vi "OAT Overall Level Plot (1 Channel).vi"(0 "even-angle signal":cluster{"r0":dbl, "dr":dbl, "Y":dbl[]}={"r0"=0.0, "dr"=1.0, "Y"=[]} {"r0" format="%.2p"; "dr" format="%.2p"; "Y" format="%.2f"}, 1 "x-axis selection":u16(ring)=2 items=["Time", "Revolution", "RPM"], 2 "reset? (F)":bool, 5 "even-angle channel info":T3={"channel name"="", "description"="", " channel info"={"sensor sensitivity"=1000.0, "engineering units"=1, "dB reference"=1.0, "custom label"="EU", "weighting filter"=0, "pregain"=0.0}} {"channel info"."pregain" format="%.2f"; "channel info"."weighting filter" items=["Linear", "A-weighting", "B-weighting", "C-weighting", "ITU-R 468-4", "Dolby", "CCITT", "C-message", "Wb", "Wc", "Wd", "We", "Wf", "Wh", "Wj", "Wk", "Wm", "AES17 20 kHz lowpass", "AES17 40 kHz lowpass", "AES17 20 kHz highpass", "AES17 40 kHz highpass"]; "channel info"."dB reference" format="%^.1e"; "channel info"."engineering units" items=["custom..."=0, "V"=1, "A"=21, "C"=30, "pC"=31, "s"=32, "-"=29, "Pa"=2, "N"=20, "g"=3, "m/s^2"=4, "m/s"=5, "m"=6, "mm/s"=12, "mm"=13, "micron/s"=14, "micron"=15, "in/s^2"=7, "in/s"=8, "in"=9, "mil/s"=10, "mil"=11, "rad/s^2"=16, "rad/s"=17, "rad"=18, "deg/s^2"=26, "deg/s"=27, "deg"=28, "RPM"=22, "cycle/s^2"=23, "Hz"=24, "cycle"=25, "strain"=19]; "channel info"."sensor sensitivity" format="%#_5f"}, 7 "even-angle position info":T1, 9 "dB on? (F)":bool, 11 "error in (no error)":errorcluster, 12 "integration revolution":dbl=1.0) -> (4 "overall level":cluster{"time/rev/rpm":dbl[], "level":dbl[]}, 6 "unit labels":T2, 8 "level position info":T1, 15 "error out":errorcluster)   [LabVIEW 2017, in "SoundVib_OrderTracking.lvlib"]
doc: "Computes the root-mean-square (RMS) level of the <B>even-angle signal</B> and generates an XY graph as the output. Wire data to the <B>even-angle signal</B> input to determine the polymorphic instance to use or manually select the instance."
uses:
  <vilib>/addons/Sound and Vibration/Order Analysis/Resample Order Tracking/SoundVib_OrderTracking.lvlib
  <vilib>/addons/Sound and Vibration/Order Analysis/Misc/OAT Position Info.ctl
  <vilib>/addons/_NISVFA/_Shared subVIs/Controls/svc_Resampled Channel Info.ctl
  <vilib>/addons/_NISVFA/_Shared subVIs/Controls/svc_Channel Info.ctl
  <vilib>/addons/_NISVFA/_Shared subVIs/Controls/svc_Engineering Units Text Ring.ctl
  <vilib>/addons/_NISVFA/_Shared subVIs/Controls/svc_Weighting Filter Text Ring.ctl
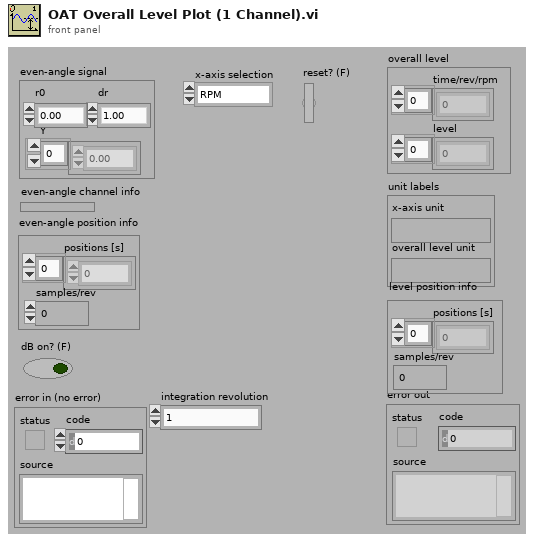
[diagram p1: front panel]
types:
  T1 = typedef "OAT Position Info.ctl" = cluster{"positions [s]":dbl[], "samples/rev":dbl}
  T2 = cluster{"x-axis unit":string, "overall level unit":string}
  T3 = typedef "svc_Resampled Channel Info.ctl" = cluster{"channel name":string, "description":string, " channel info":T4}
  T4 = typedef "svc_Channel Info.ctl" = cluster{"sensor sensitivity":dbl, "engineering units":T5, "dB reference":dbl, "custom label":string, "weighting filter":T6, "pregain":dbl}
  T5 = typedef "svc_Engineering Units Text Ring.ctl" = u16
  T6 = typedef "svc_Weighting Filter Text Ring.ctl" = u16
  T7 = cluster{"x-axis unit":string, "overall level unit":string}[]
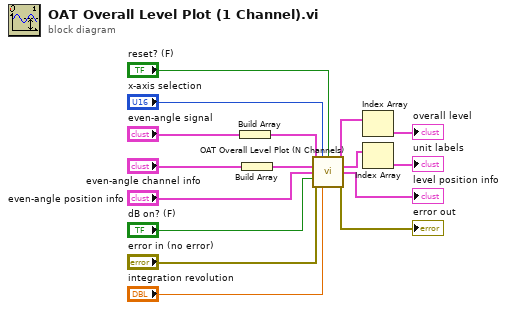
[diagram p0: block diagram]
diagram:
  n1 = Build Array("even-angle signal") -> (w3:cluster{"r0":dbl, "dr":dbl, "Y":dbl[]}[])
  n2 = Build Array("even-angle channel info") -> (w1:T3[])
  n3 = call <vilib>:"OAT Overall Level Plot (N Channels).vi"("even-angle signals"=w3, "x-axis selection"="x-axis selection", "reset? (F)"="reset? (F)", "even-angle channel info"=w1, "even-angle position info"="even-angle position info", "dB on? (F)"="dB on? (F)", "error in (no error)"="error in (no error)", "integration revolution"="integration revolution") -> ("overall levels"=w7:cluster{"time/rev/rpm":dbl[], "level":dbl[]}[], "unit labels"=w6:T7, "level position info"=→"level position info":T1, "error out"=→"error out":errorcluster)  [unwired: 4 in]
  n4 = Index Array(array=w7) -> (element=→"overall level":cluster{"time/rev/rpm":dbl[], "level":dbl[]})  [unwired: 1 in]
  n5 = Index Array(array=w6) -> (element=→"unit labels":T2)  [unwired: 1 in]
